vi "Add to Graph.vi"(0 "Value":string[][](array[string]), 1 "Current Step ID":i32, 2 "Test Table":refnum<vi>) -> ()   [LabVIEW 2010]
uses:
  <vilib>/Utility/miscctls.llb/LVRowAndColumnTypeDef.ctl
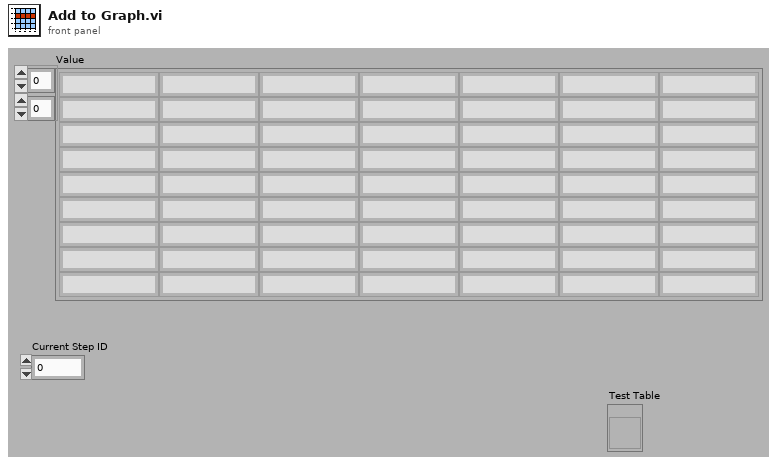
[diagram p1: front panel]
types:
  T1 = typedef "LVRowAndColumnTypeDef.ctl" = cluster{"Row":i32, "Column":i32}
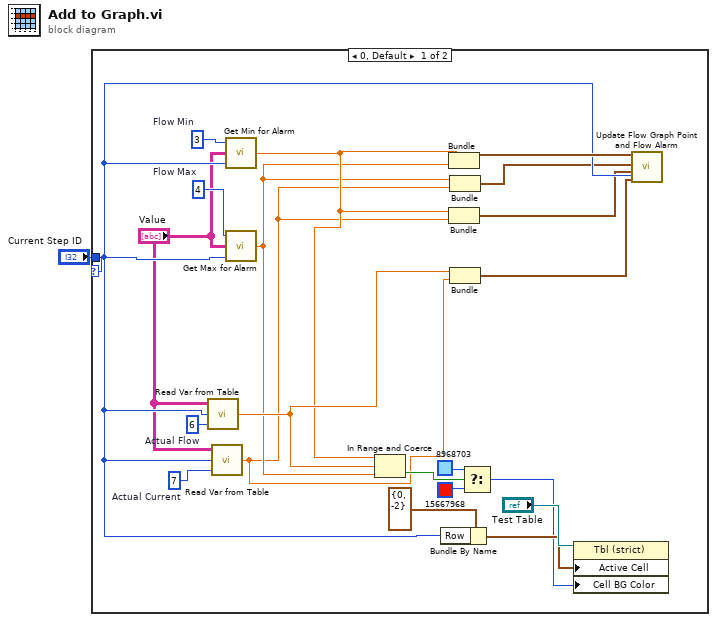
[diagram p0: block diagram]
diagram:
  n1 = case shown="0, Default" "Current Step ID" {
    tunnel: "Current Step ID" -> [w11 _]
    frame 0, Default {
      w8 = 6  # Actual Flow
      w10 = 7  # Actual Current
      w14 = 4  # Flow Max
      w15 = 3  # Flow Min
      n2 = call "Read Var from Table.vi"("VAR Column Index"=w8, "Current Step ID"=w11, "Value"="Value") -> ("Numeric"=w12:dbl)
      n3 = call "Read Var from Table.vi"("VAR Column Index"=w10, "Current Step ID"=w11, "Value"="Value") -> ("Numeric"=w5:dbl)
      n4 = call "Get Min for Alarm.vi"("Current Step Index"=w11, "Test Table"="Value", "Column Index for Min"=w15) -> ("Min"=w7:dbl)
      n5 = call "Get Max for Alarm.vi"("Current Step Index"=w11, "Test Table"="Value", "Column Index for Max"=w14) -> ("Min"=w6:dbl)
      n6 = In Range and Coerce(upper limit=w7, x=w12, lower limit=w6) -> (In Range?=w19:bool)  [unwired: 1 out]
      n7 = Bundle By Name(cluster=T1 {"Row"=0, "Column"=-2} ("Active Cell:Active Cell"), "Row"=w11) -> (w20:T1)
      n8 = Bundle("Min"=w7, "Min"=w6) -> (w13:cluster{"Min":dbl, "Min":dbl})  [unwired: 1 in]
      n9 = Bundle("Min"=w7, "Numeric"=w5) -> (w4:cluster{"Min":dbl, "Numeric":dbl})  [unwired: 1 in]
      n10 = Bundle("Min"=w6, "Numeric"=w5) -> (w3:cluster{"Min":dbl, "Numeric":dbl})  [unwired: 1 in]
      n11 = Bundle("Numeric"=w12, "Numeric"=w5) -> (w2:cluster{"Numeric":dbl, "Numeric":dbl})  [unwired: 1 in]
      n12 = Select(t=u32 8968703 ("Color Box"), s=w19, f=u32 15667968 ("Color Box")) -> (s? t:f=w16:u32)
      n13 = property class="Tbl (strict)"(reference="Test Table", "Active Cell"=w20, "Cell BG Color"=w16) -> ()  [unwired: 1 in, 2 out]
      n14 = call "Update Flow Graph Point and Flow Alarm.vi"("Current Step ID"=w11, "Actual Flow vs Current"=w2, "Low Flow Limit vs Current"=w4, "High Flow Limit vs Current"=w3, "Max and Min Flow"=w13) -> ()  [unwired: 2 in]
    }
    frame -1 {
    }
  }
